vi "Error Processor.vi"(8 "error in (no error)":errorcluster, 11 "DAQ Manager in":refnum<class "DAQ Manager.lvclass">) -> (0 "error out":errorcluster, 3 "DAQ Manager out":refnum<class "DAQ Manager.lvclass">)   [LabVIEW 2020, in "DAQ Manager.lvlib" / "DAQ Manager.lvclass"]
doc: "Use this VI to process all the error that are solvable inside this specific uService. Whatever is not possible to process, let it leave this VI and it will be processed by the Error Manager of the Distributed System."
uses:
  DAQ Manager.lvclass
  Father of all uServices/Father of all uServices/Father of all uServices.lvclass
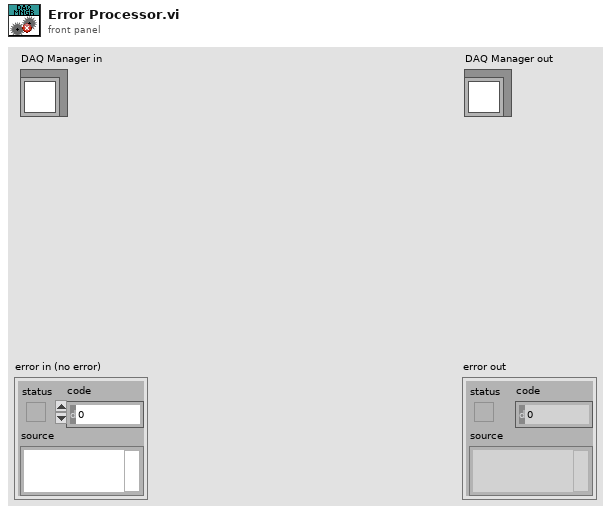
[diagram p1: front panel]
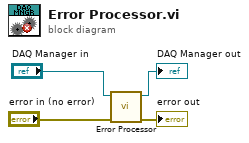
[diagram p0: block diagram]
diagram:
  n1 = call-parent "Error Processor.vi"("error in (no error)"="error in (no error)", "Father of all uServices in"="DAQ Manager in") -> ("error out"=→"error out":errorcluster, "Father of all uServices out"=→"DAQ Manager out":refnum<class "DAQ Manager.lvclass">)  [unwired: 8 in]
